vi "MarkersCoords.vi"(8 "error in (no error)":errorcluster, 9 "Markers Name":string[](array[string]), 10 "Subject Name":string, 11 ".NET Refnum in":refnum<k24>) -> (0 "error out":errorcluster, 1 "Are Markers Occluded Flags":bool[](array[boolean]), 2 "Markers Coords":dbl[][](array[numeric]), 3 ".NET Reference out":refnum<k24>)   [LabVIEW 2024]
uses:
  C:/Users/ROAR/Documents/Rob Motor Assessment stuff/Labview/RobUST_3D_with_Unity_Control_PXI_Low_Level_Only_Streamlined/Vicon_files/ViconDataStreamSDK_DotNET.dll
  Vicon_files/ViconDataStreamSDK_DotNET.dll
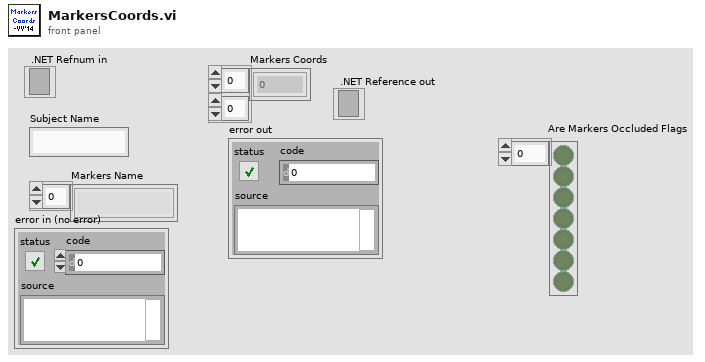
[diagram p1: front panel]
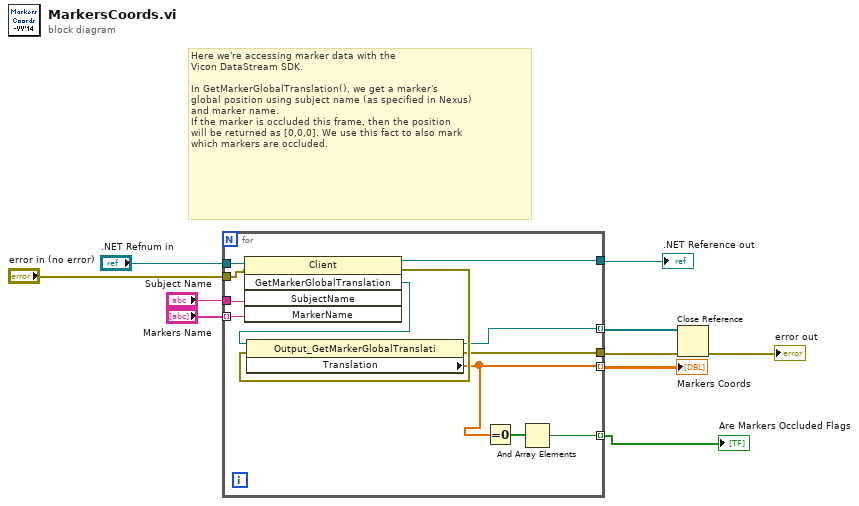
[diagram p0: block diagram]
diagram:
  # "Here we're accessing marker data with the \nVicon DataStream SDK. \n\nIn GetMarkerGlobalTranslation(), we get a marker's\nglobal position using subject name (as specified in Nexus)\nand marker name.\nIf the marker is occluded this frame, then the position\nwill be returned as [0,0,0]. We use this fact to also mark\nwhich markers are occluded."
  n1 = for {
    tunnel: ".NET Refnum in" -> [w21]
    tunnel: "Subject Name" -> [w20]
    tunnel: [w13] -> w7 mode=indexing
    tunnel: "Markers Name" -> [w19] mode=indexing
    tunnel: [w18] -> w6
    tunnel: "error in (no error)" -> [w17]
    tunnel: [w15] -> w3 mode=indexing
    tunnel: [w14] -> w2
    tunnel: [w11] -> w1 mode=indexing
    n2 = invoke class="Client" method="GetMarkerGlobalTranslation"(reference=w21, error in=w17, "SubjectName"=w20, "MarkerName"=w19) -> (reference out=w18:refnum<k24>, error out=w16:errorcluster, "GetMarkerGlobalTranslation"=w22:refnum<k24>)  [unwired: 1 in, 2 out]
    n3 = property class="Output_GetMarkerGlobalTranslati"(reference=w22, error in=w16) -> (reference out=w15:refnum<k24>, error out=w14:errorcluster, "Translation"=w13:dbl[])
    n4 = Equal To 0?(x=w13) -> (x = 0?=w12:bool[])
    n5 = And Array Elements(Boolean array=w12) -> (logical AND=w11:bool)
  }
  "Markers Coords" <- w7
  ".NET Reference out" <- w6
  "Are Markers Occluded Flags" <- w1
  n6 = Close Reference(reference=w3, error in (no error)=w2) -> (error out=→"error out":errorcluster)
